vi "VISA_Read_8CH-1graph.vi"() -> ()   [LabVIEW 2019]
uses:
  <vilib>/Instr/_visa.llb/VISA Configure Serial Port (Instr).vi
panel:
  out "Status Serial":errorcluster
  out "Plot 0":dbl[][](graph)
  out "Buffer Array":dbl[](array[numeric])
  in  "baud rate (9600)":u32=115200
  in  "data bits (8)":u8=8 min=5 max=8 step=1
  out "Status Read":errorcluster
  out "Read Buffer":string
  in  "Stop Read":bool
  in  "Start Read":bool
  in  "VISA resource name":refnum<visa-resource-name>
  # "Controle da porta Serial USB"
  # "Controle da Leitura"
  # "Log de Erros"
  # "Resultado da Leitura"
  # "CH1          CH2          CH3          CH4          CH5          CH6          CH7          CH8          CH9         CH10        CH11         CH12        CH13        CH14       CH15        CH16"
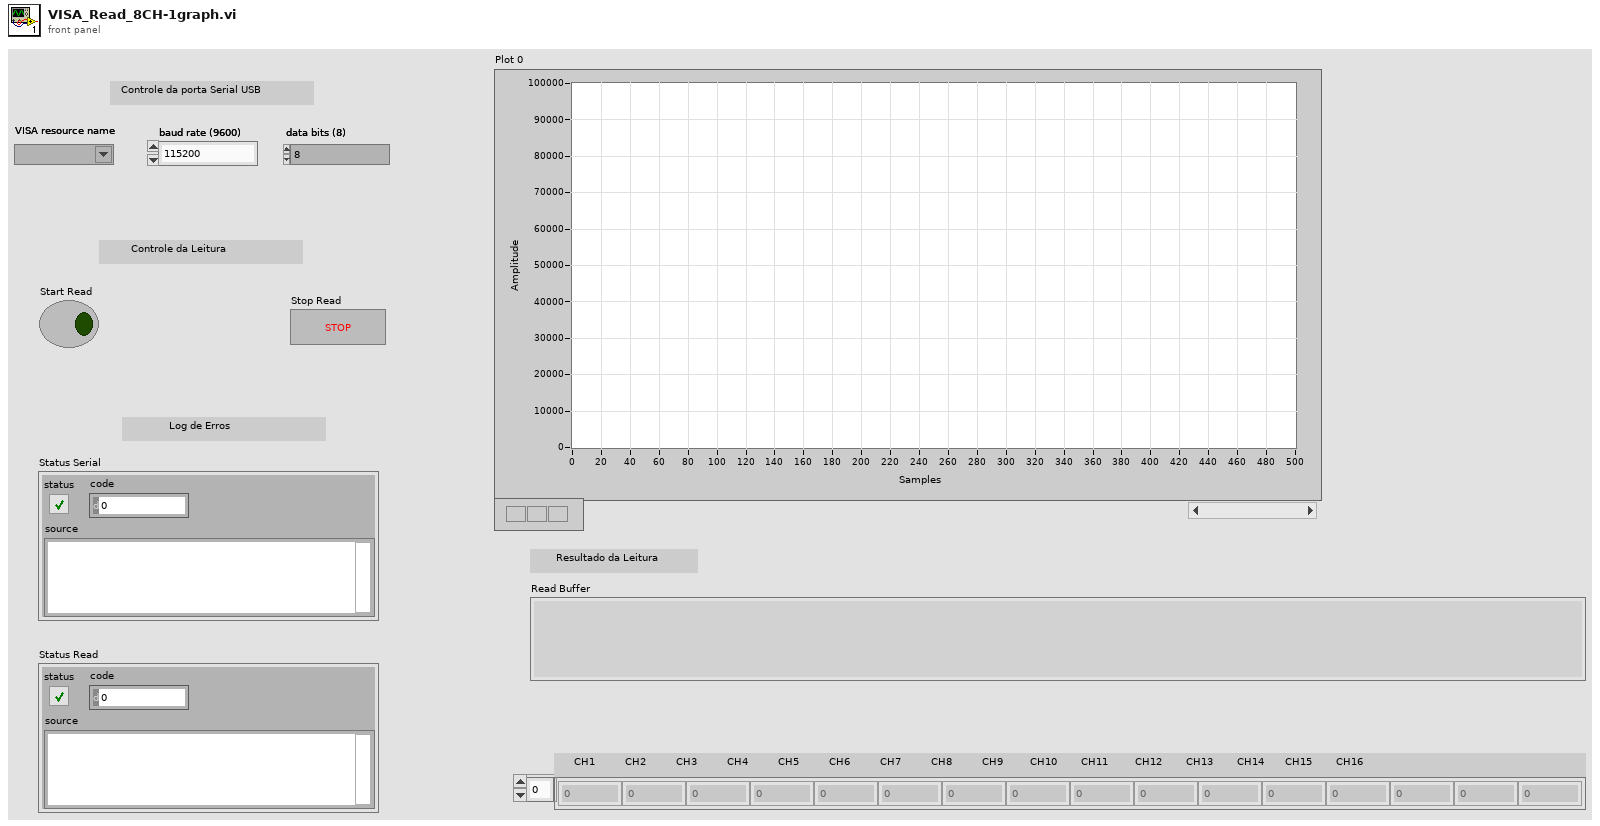
[diagram p1: front panel]
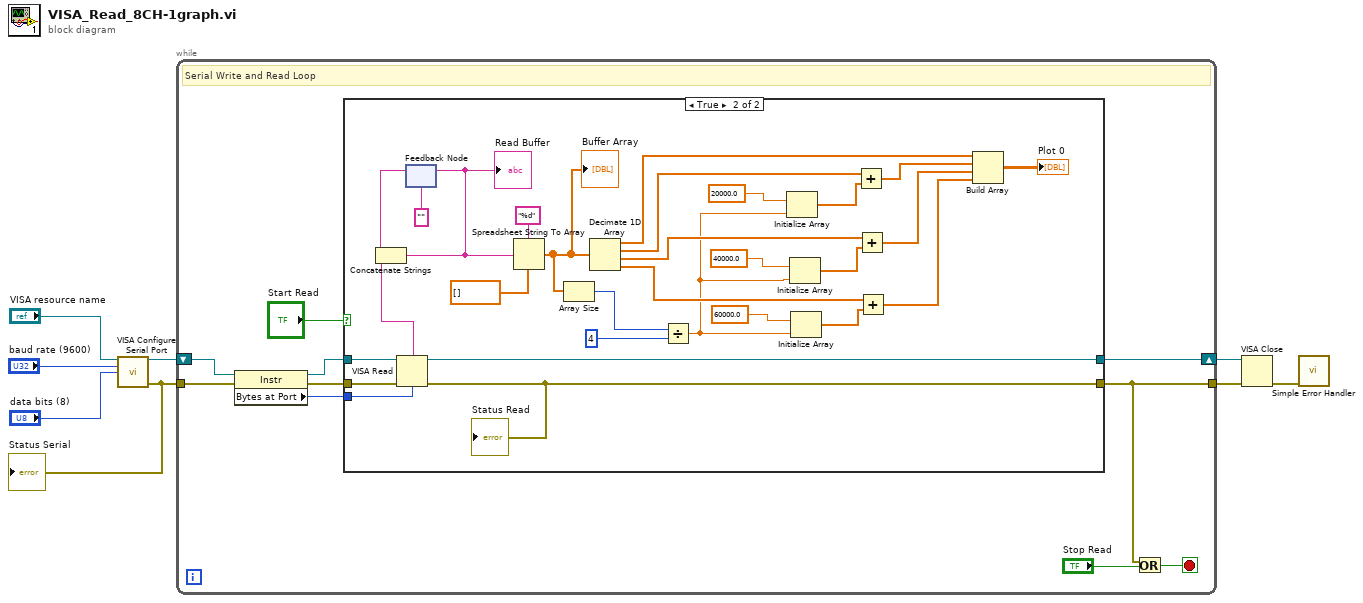
[diagram p0: block diagram]
diagram:
  n1 = call-poly "VISA Configure Serial Port"("VISA resource name"="VISA resource name", "baud rate (9600)"="baud rate (9600)", "data bits (8)"="data bits (8)") -> ("VISA resource name out"=w6:refnum<visa-resource-name>, "error out"=w1:errorcluster)  [unwired: 11 in]
  "Status Serial" <- w1
  n2 = while {
    tunnel: w1 -> [w12]
    tunnel: [w16] -> w7
    shift-right: [w15] -> w5
    shift-left: w6 -> [w13]
    stop <- w14 stop-if-true
    # "Serial Write and Read Loop"
    n3 = property class="Instr"(reference=w13, error in=w12) -> (reference out=w9:refnum<visa-resource-name>, error out=w10:errorcluster, "Bytes at Port"=w11:u32)
    n4 = case shown="True" "Start Read" {
      tunnel: [w19 w49] -> w16
      tunnel: [w20 w46] -> w15
      tunnel: w11 -> [_ w42]
      tunnel: w9 -> [w20 w41]
      tunnel: w10 -> [w19 w40]
      frame False {
      }
      frame True {
        n5 = VISA Read(VISA resource name=w41, byte count=w42, error in (no error)=w40) -> (VISA resource name out=w46:refnum<visa-resource-name>, read buffer=w48:string, error out=w49:errorcluster)  [unwired: 1 out]
        "Status Read" <- w49
        n6 = feedback #1("") -> (w43:string)
        n7 = Concatenate Strings(w43, w48) -> (w45:string)
        "Read Buffer" <- w45
        n8 = feedback-in #1(w45) -> ()
        n9 = Spreadsheet String To Array(format string="%d", spreadsheet string=w45, array type (2D Dbl)=dbl[] []) -> (array=w31:dbl[])  [unwired: 1 in]
        "Buffer Array" <- w31
        n10 = Array Size(array=w31) -> (size(s)=w30:i32)
        n11 = Decimate 1D Array(w31) -> (w35:dbl[], w38:dbl[], w37:dbl[], w36:dbl[])
        n12 = Divide(x=w30, y=4) -> (x/y=w22:dbl)
        n13 = Initialize Array(20000.0 ("element"), w22) -> (w26:dbl[])
        n14 = Initialize Array(40000.0 ("element"), w22) -> (w25:dbl[])
        n15 = Initialize Array(60000.0 ("element"), w22) -> (w24:dbl[])
        n16 = Add(x=w38, y=w26) -> (x+y=w34:dbl[])
        n17 = Add(x=w37, y=w25) -> (x+y=w33:dbl[])
        n18 = Add(x=w36, y=w24) -> (x+y=w32:dbl[])
        n19 = Build Array(w35, w34, w33, w32) -> (→"Plot 0":dbl[][])
      }
    }
    n20 = Or(x=w16, y="Stop Read") -> (x .or. y?=w14:bool)
  }
  n21 = VISA Close(VISA resource name=w5, error in (no error)=w7) -> (error out=w4:errorcluster)
  n22 = call <vilib>:"Simple Error Handler.vi"("error in (no error)"=w4) -> ()  [unwired: 4 in, 5 out]
